vi "Read Voltage.vi"() -> ()   [LabVIEW 2020]
uses:
  Classes/Generic DAQ/Generic DAQ.lvclass
  Classes/DAQmx/DAQmx.lvclass
  C:/Users/juan_/Desktop/Lab it Studio/Public/Sesiones/Sesiones/Sesion [3] 24 Mar 2025/OOP Demo/Classes/Generic DAQ/Generic DAQ.lvclass
  Classes/34972A/34972A.lvclass
panel:
  in  "Stop":bool
  out "Waveform Chart":dbl(graph)
  in  "Objects":enum16{"Sim", "DAQmx", "34972A"}(ring)
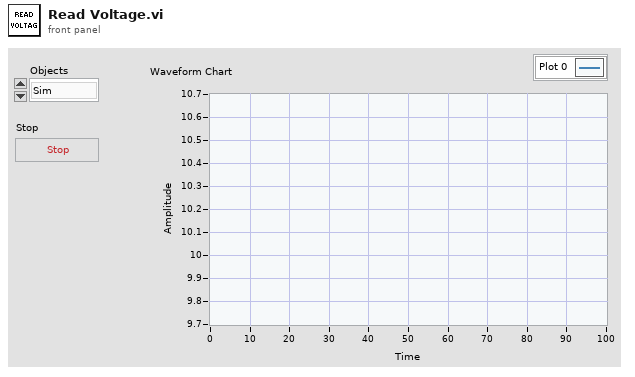
[diagram p1: front panel]
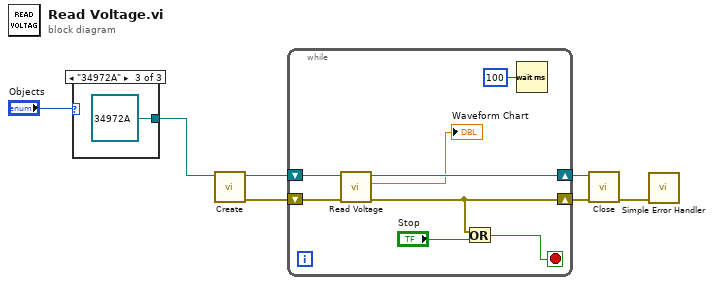
[diagram p0: block diagram]
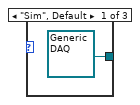
[diagram p2: hidden frame]
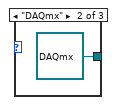
[diagram p3: hidden frame]
diagram:
  n1 = case shown="\"34972A\"" "Objects" {
    tunnel: [refnum<class "Generic DAQ.lvclass"> refnum ("Generic DAQ.lvclass") refnum<class "DAQmx.lvclass"> refnum ("DAQmx.lvclass") refnum<class "34972A.lvclass"> refnum ("34972A.lvclass")] -> w6
    frame "Sim", Default {
    }
    frame "DAQmx" {
    }
    frame "34972A" {
    }
  }
  n2 = call-dynamic "Create.vi"("Generic DAQ in"=w6) -> ("error out"=w2:errorcluster, "Generic DAQ out"=w5:refnum<class "Generic DAQ.lvclass">)  [unwired: 9 in]
  n3 = while {
    shift-right: [w17] -> w4
    shift-left: w5 -> [w18]
    shift-right: [w13] -> w3
    shift-left: w2 -> [w16]
    stop <- w11 stop-if-true
    n4 = call-dynamic "Read Voltage.vi"("error in (no error)"=w16, "Generic DAQ in"=w18) -> ("error out"=w13:errorcluster, "Voltage"=→"Waveform Chart":dbl, "Generic DAQ out"=w17:refnum<class "Generic DAQ.lvclass">)  [unwired: 7 in]
    n5 = Or(x=w13, y="Stop") -> (x .or. y?=w11:bool)
    n6 = Wait (ms)(milliseconds to wait=u32 100) -> ()  [unwired: 1 out]
  }
  n7 = call-dynamic "Close.vi"("error in (no error)"=w3, "Generic DAQ in"=w4) -> ("error out"=w1:errorcluster)  [unwired: 8 in, 1 out]
  n8 = call <vilib>:"Simple Error Handler.vi"("error in (no error)"=w1) -> ()  [unwired: 4 in, 5 out]
